vi "Swerve Controller.vi"(8 "error in":errorcluster) -> ()   [LabVIEW 2023]
doc: "This VI executes continuously carrying out the current operation and responding to updates or new operations. It will often contain the timing or control code that is difficult to place directly in TeleOp. This VI generally opens all sensors and motors and isolates the rest of the robot code from knowing how the operations are carried out."
uses:
  <vilib>/Rock Robotics/WPI/Framework/Completion Status.ctl
  Swerve Setpoints.ctl
  Swerve Operations.ctl
  <vilib>/Rock Robotics/WPI/ThirdParty/JAS_Junk/TrajLib/TypeDef/CHASSIS_SPEEDS.ctl
  <vilib>/Rock Robotics/WPI/ThirdParty/JAS_Junk/TrajLib/Trajectory_Library.lvlib
  <vilib>/Rock Robotics/Network Tables/NT Write Boolean.vi
panel:
  in  "Interactive Values":T1 {"CHASSIS"."vOmega" format="%10.3f"; "CHASSIS"."vY" format="%10.3f"; "CHASSIS"."vX" format="%10.3f"}
  out "Current\nCmd":string
  in  "Buttons":cluster{"Execute Cmd":bool, "Abort Cmd":bool}
  out "Command Timing":cluster{"Start Time (ms)":u32, "Iterations":i32}
  out "Status":T4
  # "Tip: It may be helpful to observe inputs and sensor values.\nYou may also want to display tuning or debugging controls."
  # "Interactive Command: You may fill in the settings for a command\nand schedule it with the Execute button. You can observe and abort\nany command while fine tuning the code for the controller."
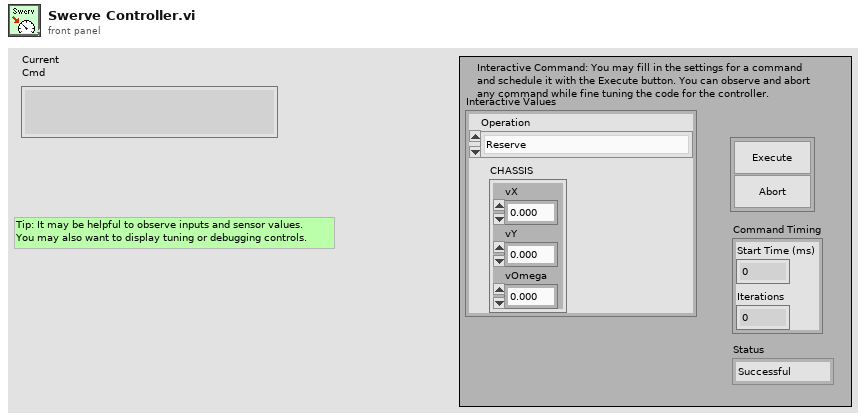
[diagram p1: front panel]
types:
  T1 = typedef "Swerve Setpoints.ctl" = cluster{"Operation":T2, "CHASSIS":T3}
  T2 = typedef "Swerve Operations.ctl" = enum16{"Reserve", "Read Current", "Immediate", "Joystick Drive"}
  T3 = typedef "Trajectory_Library.lvlib/CHASSIS_SPEEDS.ctl" = cluster{"vX":dbl, "vY":dbl, "vOmega":dbl}
  T4 = typedef "Completion Status.ctl" = enum16{"Successful", "Aborted", "Incomplete"}
  T5 = typedef "Command Status Info.ctl" = cluster{"Name":string, "Status":T4, "notifier out":T6}
  T6 = typedef "Completion Notifier.ctl" = refnum<notifier>
  T7 = cluster{"Current Command":T1, "Command Timing":cluster{"Start Time (ms)":u32, "Iterations":i32}, "Command Arguments":cluster{"Command Info":T5, "Description":string, "Default Command":T1, "queue out":refnum<queue>, "Subsystem Name":string}}
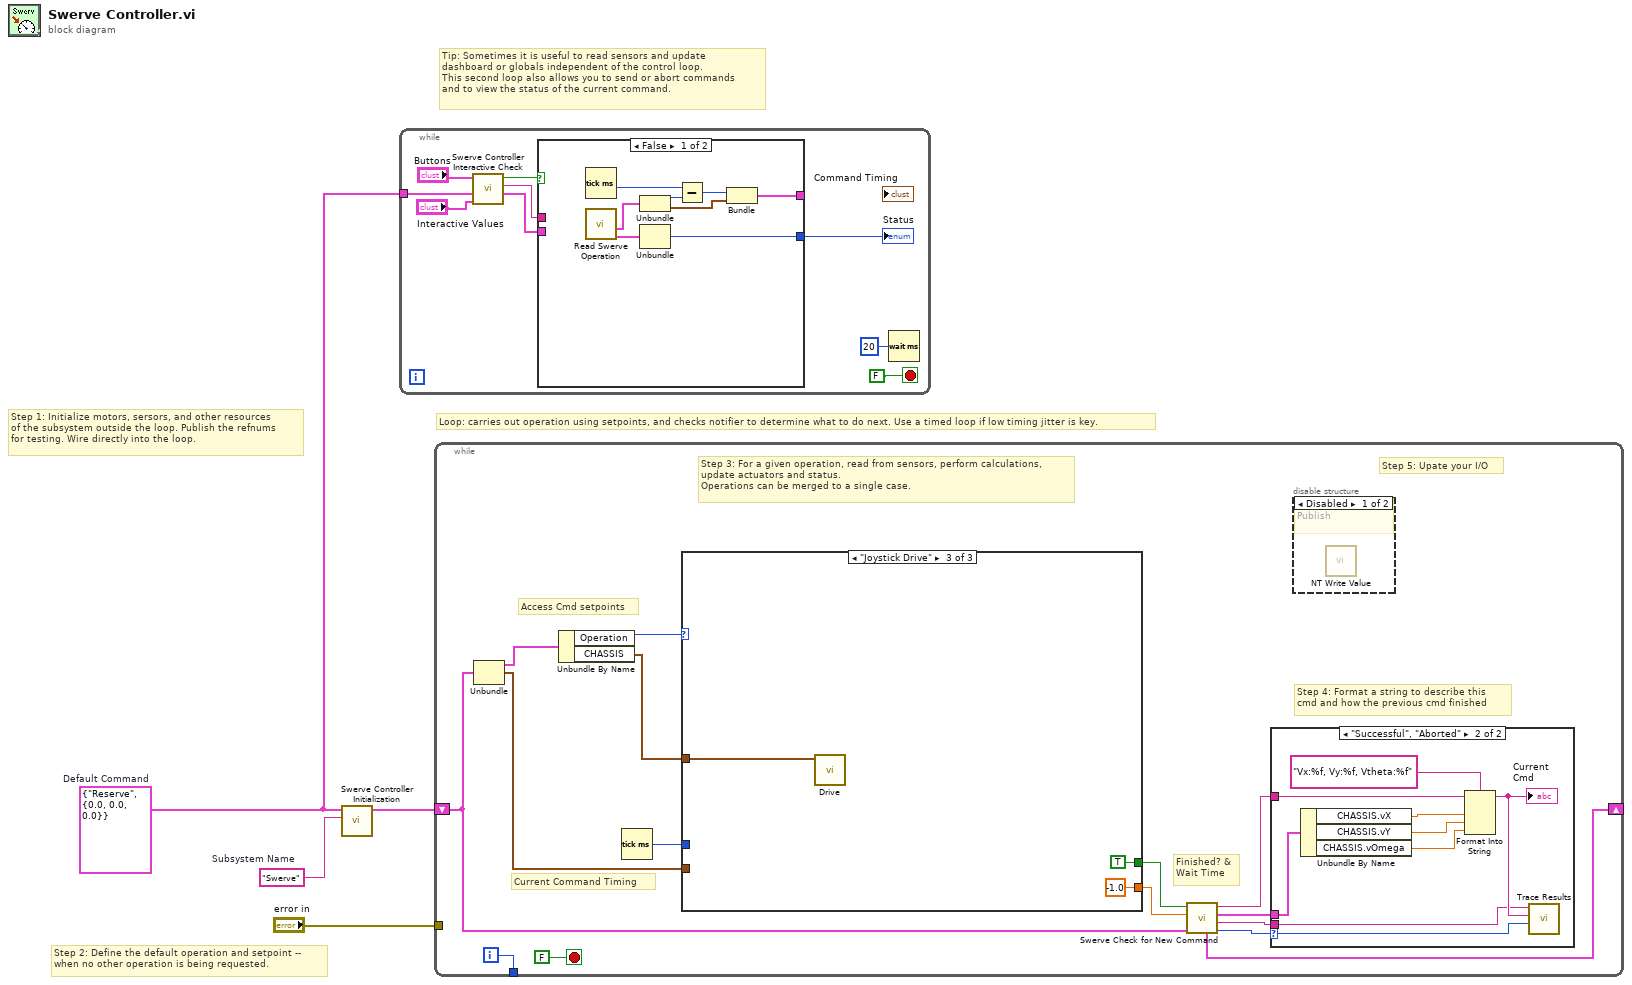
[diagram p0: block diagram]
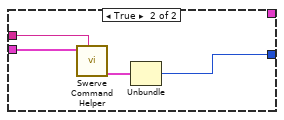
[diagram p2: hidden frame]
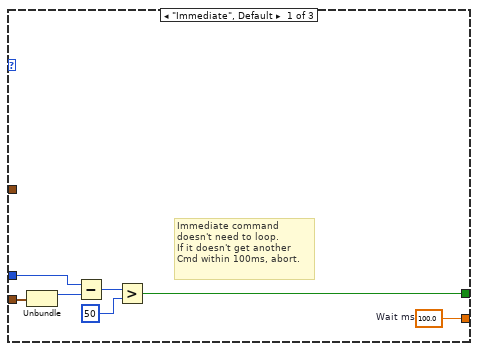
[diagram p5: hidden frame]
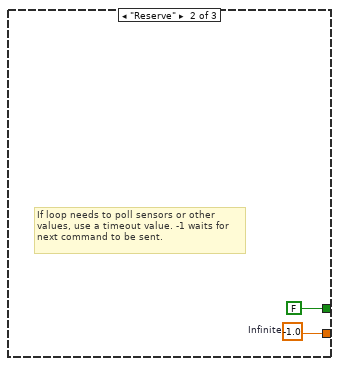
[diagram p6: hidden frame]
diagram:
  w1 = T1 {"Operation"=enum."Reserve", "CHASSIS"={"vX"=0.0, "vY"=0.0, "vOmega"=0.0}}  # Default Command
  w2 = "Swerve"  # Subsystem Name
  # "Tip: Sometimes it is useful to read sensors and update\ndashboard or globals independent of the control loop.\nThis second loop also allows you to send or abort commands\nand to view the status of the current command."
  # "Step 2: Define the default operation and setpoint --\nwhen no other operation is being requested."
  # "Step 1: Initialize motors, sersors, and other resources\nof the subsystem outside the loop. Publish the refnums\nfor testing. Wire directly into the loop."
  # "Loop: carries out operation using setpoints, and checks notifier to determine what to do next. Use a timed loop if low timing jitter is key."
  n1 = call "Swerve Controller Initialization.vi"("Subsystem Name"=w2, "Default Command"=w1) -> ("Current Command"=w3:T7)  [unwired: 9 in]
  n2 = while {
    tunnel: w1 -> [w10]
    stop <- FALSE stop-if-true
    n3 = call "Swerve Controller Interactive Check.vi"("Interactive Command in"="Interactive Values", "Default Command"=w10, "Buttons"="Buttons") -> ("Interactive Command out"=w7:T1, "Trace String"=w8:string, "Schedule"=w9:bool)  [unwired: 6 in]
    n4 = case shown="False" w9 {
      tunnel: [w21 w25] -> w6
      tunnel: w7 -> [_ w23]
      tunnel: [w17 _] -> _
      tunnel: w8 -> [_ w24]
      frame False {
        n5 = Tick Count (ms)() -> (millisecond timer value=w16:u32)
        n6 = call "Read Swerve Operation.vi"() -> ("Command Info"=w14:T5, "SubSystem Data"=w15:T1)  [unwired: 9 in, 1 out]
        n7 = Unbundle(w15) -> ("Operation"=w20:T2, "CHASSIS"=w18:T3)
        n8 = Unbundle(w14) -> ("Status"=w21:T4)  [unwired: 2 out]
        n9 = Subtract(x=w16, y=w20) -> (x-y=w19:u32)
        n10 = Bundle(w19, "CHASSIS"=w18) -> (w17:cluster{u32, "CHASSIS":T3})  [unwired: 1 in]
      }
      frame True {
        n11 = call "Swerve Command Helper.vi"("Description"=w24, "SubSystem Data"=w23) -> ("Command Info Out"=w22:T5)  [unwired: 7 in, 2 out]
        n12 = Unbundle(w22) -> ("Status"=w25:T4)  [unwired: 2 out]
      }
    }
    "Status" <- w6
    n13 = Wait (ms)(milliseconds to wait=u32 20) -> ()  [unwired: 1 out]
  }
  n14 = while {
    shift-right: [w34] -> _
    shift-left: w3 -> [w27]
    tunnel: [w39] -> _
    tunnel: "error in" -> [_]
    i -> [w39]
    stop <- FALSE stop-if-true
    # "Step 5: Upate your I/O"
    # "Step 4: Format a string to describe this\ncmd and how the previous cmd finished"
    # "Current Command Timing"
    # "Access Cmd setpoints"
    # "Finished? &\nWait Time"
    # "Step 3: For a given operation, read from sensors, perform calculations,\nupdate actuators and status.\nOperations can be merged to a single case."
    n15 = Unbundle(w27) -> ("Current Command"=w38:T1, "Command Timing"=w35:cluster{"Start Time (ms)":u32, "Iterations":i32})  [unwired: 1 out]
    n16 = Unbundle By Name(w38) -> ("Operation"=w37:T2, "CHASSIS"=w26:T3)
    n17 = Tick Count (ms)() -> (millisecond timer value=w36:u32)
    n18 = case shown="\"Joystick Drive\"" w37 {
      tunnel: [w56 w58 -1.0 ("Infinite")] -> w32
      tunnel: [w50 FALSE ("ignore previous (F)") TRUE ("ignore previous (F)")] -> w33
      tunnel: w35 -> [w52 _ _]
      tunnel: w36 -> [w51 _ _]
      tunnel: w26 -> [_ _ w59]
      frame "Immediate", Default {
        w56 = 100.0  # Wait ms
        # "Immediate command\ndoesn't need to loop.\nIf it doesn't get another\nCmd within 100ms, abort."
        n19 = Unbundle(w52) -> ("Start Time (ms)"=w55:u32)  [unwired: 1 out]
        n20 = Subtract(x=w51, y=w55) -> (x-y=w54:u32)
        n21 = Greater?(x=w54, y=u8 50 ("Left Motor")) -> (0:w50:bool)
      }
      frame "Reserve" {
        w58 = -1.0  # Infinite
        # "If loop needs to poll sensors or other\nvalues, use a timeout value. -1 waits for\nnext command to be sent."
      }
      frame "Joystick Drive" {
        n22 = call "Drive.vi"("CHASSIS"=w59) -> ()  [unwired: 9 in, 2 out]
      }
    }
    n23 = call "Swerve Check for New Command.vi"("Current Command"=w27, "Wait time (ms)"=w32, "Finished?"=w33) -> ("Completion"=w28:T4, "Subsystem Name"=w29:string, "Current Command"=w30:T1, "Initial Trace String"=w31:string, "NextCommand"=w34:T7)  [unwired: 4 in]
    n24 = case shown="\"Successful\", \"Aborted\"" w28 {
      selector: w28 -> [_ w49]
      tunnel: w31 -> [_ w45]
      tunnel: w30 -> [_ w46]
      tunnel: w29 -> [_ w42]
      frame "Incomplete", Default {
        # "Continuing current command"
      }
      frame "Successful", "Aborted" {
        # "Report and setup for next command"
        n25 = Unbundle By Name(w46) -> ("CHASSIS.vX"=w48:dbl, "CHASSIS.vY"=w43:dbl, "CHASSIS.vOmega"=w41:dbl)
        n26 = Format Into String(format string="Vx:%f, Vy:%f, Vtheta:%f", initial string=w45, w48, w43, w41) -> (resulting string=w44:string)  [unwired: 1 in, 1 out]
        "Current\nCmd" <- w44
        n27 = call <vilib>:"Trace Results.vi"("Status of previous command"=w49, "Description"=w44, "Subsystem"=w42) -> ()  [unwired: 9 in]
      }
    }
    n28 = disable-structure shown="Disabled" {
      frame Disabled {
        # "Publish"
        n29 = call-poly <vilib>:"NT Write Value.vi"() -> ()  [unwired: 11 in, 1 out]
      }
      frame Enabled {
      }
    }
  }
